vi "replFolderStructure.vi"(8 "error in (no error)":errorcluster, 11 "File to convert":path) -> (0 "error out":errorcluster, 3 "rep path":path)   [LabVIEW 2017]
doc: "Mimics the folder structure in the VI and will replicate it in the Destination Folder."
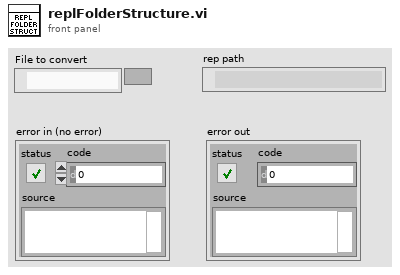
[diagram p1: front panel]
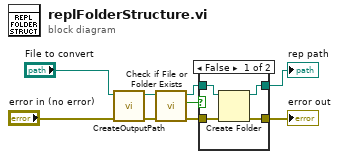
[diagram p0: block diagram]
diagram:
  n1 = call "CreateOutputPath.vi"("error in (no error)"="error in (no error)", "File to convert"="File to convert") -> ("error out"=w1:errorcluster, "appended path"=w4:path)  [unwired: 8 in]
  n2 = call <vilib>:"Check if File or Folder Exists.vi"("error in (no error)"=w1, "path"=w4) -> ("error out"=w6:errorcluster, "file or folder exists?"=w7:bool, "dup path"=w5:path)  [unwired: 7 in]
  n3 = case shown="False" w7 {
    tunnel: w5 -> [w10 w15]
    tunnel: [w13 w15] -> w8
    tunnel: w6 -> [w11 w14]
    tunnel: [w12 w14] -> w9
    frame False {
      n4 = Create Folder(path (use dialog)=w10, error in=w11) -> (created path=w13:path, error out=w12:errorcluster)  [unwired: 1 in, 1 out]
    }
    frame True {
    }
  }
  "error out" <- w9
  "rep path" <- w8
